vi "Read Data.vi"(8 "error in (no error)":errorcluster, 11 "EGG5302 in":refnum<class "EGG5302.lvclass">) -> (0 "error out":errorcluster, 2 "Data":waveform(dbl)[](array[waveform]), 3 "EGG5302 out":refnum<class "EGG5302.lvclass">)   [LabVIEW 2015, in "EGG5302.lvclass"]
uses:
  EGG5302.lvclass
  Instrument/Instrument.lvclass
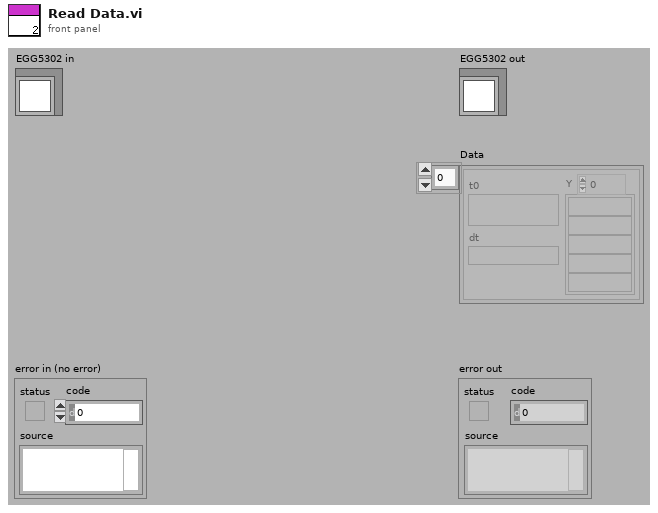
[diagram p1: front panel]
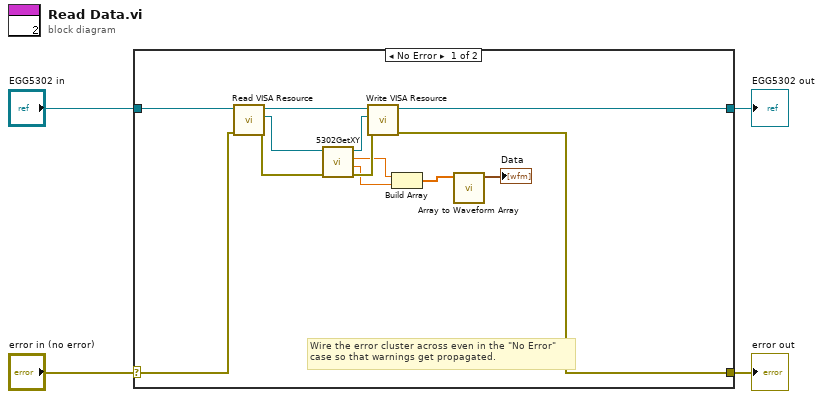
[diagram p0: block diagram]
diagram:
  n1 = case shown="No Error" "error in (no error)" {
    selector: "error in (no error)" -> [w14 w19]
    tunnel: [w9 w19] -> w3
    tunnel: [w12 w18] -> w1
    tunnel: "EGG5302 in" -> [w17 w18]
    frame No Error {
      # "Wire the error cluster across even in the \"No Error\"\ncase so that warnings get propagated."
      n2 = call "Read VISA Resource.vi"("error in (no error)"=w14, "Instrument.lvclass in"=w17) -> ("error out"=w13:errorcluster, "VISA Resource"=w15:refnum<visa-resource-name>, "Instrument.lvclass out"=w16:refnum<class "EGG5302.lvclass">)  [unwired: 7 out]
      n3 = call "5302GetXY.vi"("error in (no error)"=w13, "VISA Resource Name"=w15) -> ("error out"=w10:errorcluster, "Y"=w6:dbl, "X"=w7:dbl, "VISA Resource Name Out"=w11:refnum<visa-resource-name>)  [unwired: 1 in, 5 out]
      n4 = call "Write VISA Resource.vi"("error in (no error)"=w10, "VISA Resource"=w11, "Instrument.lvclass in"=w16) -> ("error out"=w9:errorcluster, "Instrument.lvclass out"=w12:refnum<class "EGG5302.lvclass">)  [unwired: 7 out]
      n5 = Build Array(w7, w6) -> (w8:dbl[])
      n6 = call "Array to Waveform Array.vi"("Array"=w8) -> ("Waveform"=→"Data":waveform(dbl)[])  [unwired: 10 in]
    }
    frame Error {
    }
  }
  "error out" <- w3
  "EGG5302 out" <- w1
